vi "niRFUtil WFM Add Waveforms (complex wfm).vi"(2 "Waveform 2 In":T1 {"y" format="%.2f"; "dx" format="%^.2e"; "x0" format="%^.2e"}, 3 "Waveform 1 In":T1 {"y" format="%.2f"; "dx" format="%^.2e"; "x0" format="%^.2e"}) -> (1 "Waveform Out":T1 {"y" format="%.2f"; "dx" format="%^.2e"; "x0" format="%^.2e"})   [LabVIEW 2015, in "niRFUtil.lvlib"]
doc: "(c) Copyright 2006, National Instruments, Inc. This VI may not be duplicated, sold, or distributed without written consent from National Instruments."
uses:
  niRFUtil.lvlib
  Includes/niRFUtil INC Complex Waveform.ctl
  Includes/niRFUtil INC Complex Array.ctl
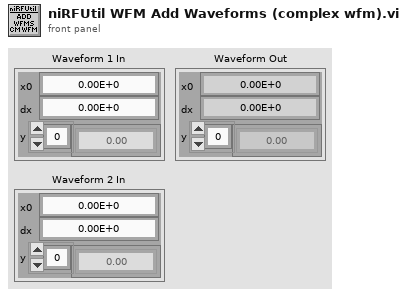
[diagram p1: front panel]
types:
  T1 = typedef "niRFUtil.lvlib/niRFUtil INC Complex Waveform.ctl" = cluster{"x0":dbl, "dx":dbl, "y":T2}
  T2 = typedef "niRFUtil.lvlib/niRFUtil INC Complex Array.ctl" = csg[]
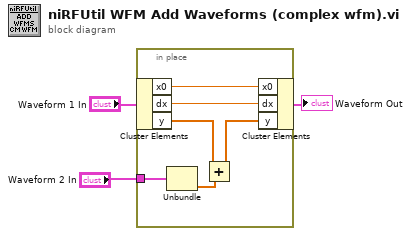
[diagram p0: block diagram]
diagram:
  n1 = in-place {
    in-place-border: "Waveform 2 In" -> [w8]
    n2 = in-place-cluster #1("Waveform 1 In") -> ("x0"=w7:dbl, "dx"=w6:dbl, "y"=w5:T2)
    n3 = Unbundle(w8) -> ("y"=w9:T2)  [unwired: 2 out]
    n4 = Add(x=w5, y=w9) -> (x+y=w4:T2)
    n5 = in-place-cluster #1("x0"=w7, "dx"=w6, "y"=w4) -> (→"Waveform Out":T1)
  }
